vi "Hardware Out - ECS-100X.vi"(11 "RT Data in":T1={"Refs"={"FPGA 1"=refnum, "FPGA 2"=refnum}, "EPT"={"MaxCAD"=0.0, "EPT Sim Enabled"=FALSE, "EPTxData"={"Sync"=FALSE, "CurrentCAD"=0.0, "Speed [RPM]"=0.0, "Config"=FALSE, "Rcvg Primary"=FALSE, "Stall"=FALSE, "Overflow"=FALSE, "Ratio Error"=FALSE, "Pattern Error"=FALSE, "Aux Warning"=FALSE, "Watchdog Error"=FALSE}}, "Raw Inputs"={"NI9752s"=[], "NI9757s"=[], "NI9411s"=[], "NI9220s"=[], "VRHalls"=[]}, "Control Inputs"={"Engine Speed [RPM]"=0.0, "Engine Status"=enum."STALLED", "Load Control \nMode"=enum."High-Idle Governor", "dt(s)"=0.0, "Number of Cylinders"=0, "Engine Displacement [cc]"=0.0, "StoichAFR"=0.0, "Q.LHV Fuel [kJ/kg]"=0.0, "BattV PSU [V]"=0.0, "12V PSU [V]"=0.0, "5V PSU [V]"=0.0, "Pedal Position [%]"=0.0, "Oil Pressure [kPa]"=0.0, "Oil Temp [C]"=0.0, "Oil Level [%]"=0.0, "Engine Coolant Temp (ECT) [C]"=0.0, "Engine Coolant Pressure [kPa]"=0.0, "Rail Pressure [bar]"=0.0, "Fuel Pressure [kPa]"=0.0, "Fuel Temp [C]"=0.0, "Vacuum Pressure [kPa]"=0.0, "Throttle Position [%]"=0.0, "Cam1 Advance [CAD]"=0.0, "Cam2 Advance [CAD]"=0.0, "Cam3 Advance [CAD]"=0.0, "Cam4 Advance [CAD]"=0.0, "CA50 Control Output [CAD]"=[], "CA50 Control Output Valid"=[], "Intake Air Temp (IAT) [C]"=0.0, "Barometric Air Pressure [kPa]"=0.0, "Intake Air Rel. Humidity [%]"=0.0, "Mass Air Flow (MAF) [kg/hr]"=0.0, "Turbo Inlet Air Pressure [kPa]"=0.0, "Turbo Inlet Air Temp [C]"=0.0, "Turbo Outlet Air Pressure [kPa]"=0.0, "Turbo Outlet Air Temp [C]"=0.0, "CAC Outlet Pressure [kPa]"=0.0, "CAC Outlet Temp [C]"=0.0, "Intake Manifold Pressure (MAP) [kPa]"=0.0, "Intake Manifold Temp (MAT) [C]"=0.0, "Exhaust Manifold Pressure [kPa]"=0.0, "Exhaust Manifold Temp [C]"=0.0, "HighP EGR Cooler Outlet Pressure [kPa]"=0.0, "HighP EGR Cooler Outlet Temp [C]"=0.0, "HighP EGR Differential Pressure [kPa]"=0.0, "HighP EGR Valve Position [%]"=0.0, "Turbo Outlet Exhaust Pressure [kPa]"=0.0, "Turbo Outlet Exhaust Temp [C]"=0.0, "VGT Position 1 [%]"=0.0, "VGT Position 2 [%]"=0.0, "Turbo Speed 1 [RPM]"=0.0, "Turbo Speed 2 [RPM]"=0.0, "LowP EGR Differential Pressure [kPa]"=0.0, "LowP EGR Valve Position [%]"=0.0, "UEGO1Lambda"=0.0, "UEGO1_Hot"=FALSE, "UEGO2Lambda"=0.0, "UEGO2_Hot"=FALSE, "Knock Intensity"=[], "Knock"=[]}, "Control Outputs"={"Pedal Desired [%]"=0.0, "MEP Desired [bar]"=0.0, "Fuel Desired [mg/cyc]"=0.0, "Intake MAP Desired [kPa]"=0.0, "Cam1 Advance Setpoint [CAD]"=0.0, "Cam2 Advance Setpoint [CAD]"=0.0, "HighP EGR Position Setpoint [%Open]"=0.0, "LowP EGR Position Setpoint [%Open]"=0.0, "Rail Pressure Setpoint [bar]"=0.0, "Wastegate1 Position Setpoint [%Open]"=0.0, "Wastegate2 Position Setpoint [%Open]"=0.0, "VGT1 Position Setpoint [%Open]"=0.0, "VGT2 Position Setpoint [%Open]"=0.0, "Throttle1 Position Setpoint [%Open]"=0.0, "Throttle2 Position Setpoint [%Open]"=0.0, "TurboBPV Position Setpoint [%Open]"=0.0, "Spark Dwells [msec]"=[], "Spark Timings [DBTDC]"=[], "PFI Quantities [mg/inj]"=[], "PFI Timings [DBTDC]"=[], "DI Quantities [mg/inj]"=[], "DI Timings [DBTDC]"=[]}, "Raw Outputs"={"9751-1"={"DI1"={"Window_Start (DBTDC)"=0.0, "Window_End (DBTDC)"=0.0, "Enable_Inj1"=FALSE, "Duration_Inj1 (msec)"=0.0, "Timing_Inj1 (DBTDC)"=0.0, "Enable_Inj2"=FALSE, "Duration_Inj2 (msec)"=0.0, "Timing_Inj2 (DBTDC)"=0.0, "Enable_Inj3"=FALSE, "Duration_Inj3 (msec)"=0.0, "Timing_Inj3 (DBTDC)"=0.0, "Enable_Inj4"=FALSE, "Duration_Inj4 (msec)"=0.0, "Timing_Inj4 (DBTDC)"=0.0, "Enable_Inj5"=FALSE, "Duration_Inj5 (msec)"=0.0, "Timing_Inj5 (DBTDC)"=0.0}, "DI2"={"Window_Start (DBTDC)"=0.0, "Window_End (DBTDC)"=0.0, "Enable_Inj1"=FALSE, "Duration_Inj1 (msec)"=0.0, "Timing_Inj1 (DBTDC)"=0.0, "Enable_Inj2"=FALSE, "Duration_Inj2 (msec)"=0.0, "Timing_Inj2 (DBTDC)"=0.0, "Enable_Inj3"=FALSE, "Duration_Inj3 (msec)"=0.0, "Timing_Inj3 (DBTDC)"=0.0, "Enable_Inj4"=FALSE, "Duration_Inj4 (msec)"=0.0, "Timing_Inj4 (DBTDC)"=0.0, "Enable_Inj5"=FALSE, "Duration_Inj5 (msec)"=0.0, "Timing_Inj5 (DBTDC)"=0.0}, "DI3"={"Window_Start (DBTDC)"=0.0, "Window_End (DBTDC)"=0.0, "Enable_Inj1"=FALSE, "Duration_Inj1 (msec)"=0.0, "Timing_Inj1 (DBTDC)"=0.0, "Enable_Inj2"=FALSE, "Duration_Inj2 (msec)"=0.0, "Timing_Inj2 (DBTDC)"=0.0, "Enable_Inj3"=FALSE, "Duration_Inj3 (msec)"=0.0, "Timing_Inj3 (DBTDC)"=0.0, "Enable_Inj4"=FALSE, "Duration_Inj4 (msec)"=0.0, "Timing_Inj4 (DBTDC)"=0.0, "Enable_Inj5"=FALSE, "Duration_Inj5 (msec)"=0.0, "Timing_Inj5 (DBTDC)"=0.0}}, "9751-2"={"DI1"={"Window_Start (DBTDC)"=0.0, "Window_End (DBTDC)"=0.0, "Enable_Inj1"=FALSE, "Duration_Inj1 (msec)"=0.0, "Timing_Inj1 (DBTDC)"=0.0, "Enable_Inj2"=FALSE, "Duration_Inj2 (msec)"=0.0, "Timing_Inj2 (DBTDC)"=0.0, "Enable_Inj3"=FALSE, "Duration_Inj3 (msec)"=0.0, "Timing_Inj3 (DBTDC)"=0.0, "Enable_Inj4"=FALSE, "Duration_Inj4 (msec)"=0.0, "Timing_Inj4 (DBTDC)"=0.0, "Enable_Inj5"=FALSE, "Duration_Inj5 (msec)"=0.0, "Timing_Inj5 (DBTDC)"=0.0}, "DI2"={"Window_Start (DBTDC)"=0.0, "Window_End (DBTDC)"=0.0, "Enable_Inj1"=FALSE, "Duration_Inj1 (msec)"=0.0, "Timing_Inj1 (DBTDC)"=0.0, "Enable_Inj2"=FALSE, "Duration_Inj2 (msec)"=0.0, "Timing_Inj2 (DBTDC)"=0.0, "Enable_Inj3"=FALSE, "Duration_Inj3 (msec)"=0.0, "Timing_Inj3 (DBTDC)"=0.0, "Enable_Inj4"=FALSE, "Duration_Inj4 (msec)"=0.0, "Timing_Inj4 (DBTDC)"=0.0, "Enable_Inj5"=FALSE, "Duration_Inj5 (msec)"=0.0, "Timing_Inj5 (DBTDC)"=0.0}, "DI3"={"Window_Start (DBTDC)"=0.0, "Window_End (DBTDC)"=0.0, "Enable_Inj1"=FALSE, "Duration_Inj1 (msec)"=0.0, "Timing_Inj1 (DBTDC)"=0.0, "Enable_Inj2"=FALSE, "Duration_Inj2 (msec)"=0.0, "Timing_Inj2 (DBTDC)"=0.0, "Enable_Inj3"=FALSE, "Duration_Inj3 (msec)"=0.0, "Timing_Inj3 (DBTDC)"=0.0, "Enable_Inj4"=FALSE, "Duration_Inj4 (msec)"=0.0, "Timing_Inj4 (DBTDC)"=0.0, "Enable_Inj5"=FALSE, "Duration_Inj5 (msec)"=0.0, "Timing_Inj5 (DBTDC)"=0.0}}, "9751-3"={"DI1"={"Window_Start (DBTDC)"=0.0, "Window_End (DBTDC)"=0.0, "Enable_Inj1"=FALSE, "Duration_Inj1 (msec)"=0.0, "Timing_Inj1 (DBTDC)"=0.0, "Enable_Inj2"=FALSE, "Duration_Inj2 (msec)"=0.0, "Timing_Inj2 (DBTDC)"=0.0, "Enable_Inj3"=FALSE, "Duration_Inj3 (msec)"=0.0, "Timing_Inj3 (DBTDC)"=0.0, "Enable_Inj4"=FALSE, "Duration_Inj4 (msec)"=0.0, "Timing_Inj4 (DBTDC)"=0.0, "Enable_Inj5"=FALSE, "Duration_Inj5 (msec)"=0.0, "Timing_Inj5 (DBTDC)"=0.0}, "DI2"={"Window_Start (DBTDC)"=0.0, "Window_End (DBTDC)"=0.0, "Enable_Inj1"=FALSE, "Duration_Inj1 (msec)"=0.0, "Timing_Inj1 (DBTDC)"=0.0, "Enable_Inj2"=FALSE, "Duration_Inj2 (msec)"=0.0, "Timing_Inj2 (DBTDC)"=0.0, "Enable_Inj3"=FALSE, "Duration_Inj3 (msec)"=0.0, "Timing_Inj3 (DBTDC)"=0.0, "Enable_Inj4"=FALSE, "Duration_Inj4 (msec)"=0.0, "Timing_Inj4 (DBTDC)"=0.0, "Enable_Inj5"=FALSE, "Duration_Inj5 (msec)"=0.0, "Timing_Inj5 (DBTDC)"=0.0}, "DI3"={"Window_Start (DBTDC)"=0.0, "Window_End (DBTDC)"=0.0, "Enable_Inj1"=FALSE, "Duration_Inj1 (msec)"=0.0, "Timing_Inj1 (DBTDC)"=0.0, "Enable_Inj2"=FALSE, "Duration_Inj2 (msec)"=0.0, "Timing_Inj2 (DBTDC)"=0.0, "Enable_Inj3"=FALSE, "Duration_Inj3 (msec)"=0.0, "Timing_Inj3 (DBTDC)"=0.0, "Enable_Inj4"=FALSE, "Duration_Inj4 (msec)"=0.0, "Timing_Inj4 (DBTDC)"=0.0, "Enable_Inj5"=FALSE, "Duration_Inj5 (msec)"=0.0, "Timing_Inj5 (DBTDC)"=0.0}}, "9751-4"={"DI1"={"Window_Start (DBTDC)"=0.0, "Window_End (DBTDC)"=0.0, "Enable_Inj1"=FALSE, "Duration_Inj1 (msec)"=0.0, "Timing_Inj1 (DBTDC)"=0.0, "Enable_Inj2"=FALSE, "Duration_Inj2 (msec)"=0.0, "Timing_Inj2 (DBTDC)"=0.0, "Enable_Inj3"=FALSE, "Duration_Inj3 (msec)"=0.0, "Timing_Inj3 (DBTDC)"=0.0, "Enable_Inj4"=FALSE, "Duration_Inj4 (msec)"=0.0, "Timing_Inj4 (DBTDC)"=0.0, "Enable_Inj5"=FALSE, "Duration_Inj5 (msec)"=0.0, "Timing_Inj5 (DBTDC)"=0.0}, "DI2"={"Window_Start (DBTDC)"=0.0, "Window_End (DBTDC)"=0.0, "Enable_Inj1"=FALSE, "Duration_Inj1 (msec)"=0.0, "Timing_Inj1 (DBTDC)"=0.0, "Enable_Inj2"=FALSE, "Duration_Inj2 (msec)"=0.0, "Timing_Inj2 (DBTDC)"=0.0, "Enable_Inj3"=FALSE, "Duration_Inj3 (msec)"=0.0, "Timing_Inj3 (DBTDC)"=0.0, "Enable_Inj4"=FALSE, "Duration_Inj4 (msec)"=0.0, "Timing_Inj4 (DBTDC)"=0.0, "Enable_Inj5"=FALSE, "Duration_Inj5 (msec)"=0.0, "Timing_Inj5 (DBTDC)"=0.0}, "DI3"={"Window_Start (DBTDC)"=0.0, "Window_End (DBTDC)"=0.0, "Enable_Inj1"=FALSE, "Duration_Inj1 (msec)"=0.0, "Timing_Inj1 (DBTDC)"=0.0, "Enable_Inj2"=FALSE, "Duration_Inj2 (msec)"=0.0, "Timing_Inj2 (DBTDC)"=0.0, "Enable_Inj3"=FALSE, "Duration_Inj3 (msec)"=0.0, "Timing_Inj3 (DBTDC)"=0.0, "Enable_Inj4"=FALSE, "Duration_Inj4 (msec)"=0.0, "Timing_Inj4 (DBTDC)"=0.0, "Enable_Inj5"=FALSE, "Duration_Inj5 (msec)"=0.0, "Timing_Inj5 (DBTDC)"=0.0}}, "9754-1"={"ESTTL 1"={"Timing (DBTDC)"=0.0, "Dwell (ms)"=0.0}, "ESTTL 2"={"Timing (DBTDC)"=0.0, "Dwell (ms)"=0.0}, "ESTTL 3"={"Timing (DBTDC)"=0.0, "Dwell (ms)"=0.0}, "ESTTL 4"={"Timing (DBTDC)"=0.0, "Dwell (ms)"=0.0}, "ESTTL 5"={"Timing (DBTDC)"=0.0, "Dwell (ms)"=0.0}, "ESTTL 6"={"Timing (DBTDC)"=0.0, "Dwell (ms)"=0.0}, "ESTTL 7"={"Timing (DBTDC)"=0.0, "Dwell (ms)"=0.0}, "ESTTL 8"={"Timing (DBTDC)"=0.0, "Dwell (ms)"=0.0}}, "9754-2"={"ESTTL 1"={"Timing (DBTDC)"=0.0, "Dwell (ms)"=0.0}, "ESTTL 2"={"Timing (DBTDC)"=0.0, "Dwell (ms)"=0.0}, "ESTTL 3"={"Timing (DBTDC)"=0.0, "Dwell (ms)"=0.0}, "ESTTL 4"={"Timing (DBTDC)"=0.0, "Dwell (ms)"=0.0}, "ESTTL 5"={"Timing (DBTDC)"=0.0, "Dwell (ms)"=0.0}, "ESTTL 6"={"Timing (DBTDC)"=0.0, "Dwell (ms)"=0.0}, "ESTTL 7"={"Timing (DBTDC)"=0.0, "Dwell (ms)"=0.0}, "ESTTL 8"={"Timing (DBTDC)"=0.0, "Dwell (ms)"=0.0}}, "9758-1"={"LS 1"={"Enable"=FALSE, "Freq [Hz]"=0.0, "DutyCyc [%]"=0.0}, "LS 2"={"Enable"=FALSE, "Freq [Hz]"=0.0, "DutyCyc [%]"=0.0}, "LS 3"={"Enable"=FALSE, "Freq [Hz]"=0.0, "DutyCyc [%]"=0.0}, "LS 4"={"Enable"=FALSE, "Freq [Hz]"=0.0, "DutyCyc [%]"=0.0}, "PFI 1"={"Position Mode"=FALSE, "Timing (DBTDC)"=0.0, "Pulse Width (ms)"=0.0}, "PFI 2"={"Position Mode"=FALSE, "Timing (DBTDC)"=0.0, "Pulse Width (ms)"=0.0}, "PFI 3"={"Position Mode"=FALSE, "Timing (DBTDC)"=0.0, "Pulse Width (ms)"=0.0}, "PFI 4"={"Position Mode"=FALSE, "Timing (DBTDC)"=0.0, "Pulse Width (ms)"=0.0}}, "9758-2"={"LS 1"={"Enable"=FALSE, "Freq [Hz]"=0.0, "DutyCyc [%]"=0.0}, "LS 2"={"Enable"=FALSE, "Freq [Hz]"=0.0, "DutyCyc [%]"=0.0}, "LS 3"={"Enable"=FALSE, "Freq [Hz]"=0.0, "DutyCyc [%]"=0.0}, "LS 4"={"Enable"=FALSE, "Freq [Hz]"=0.0, "DutyCyc [%]"=0.0}, "PFI 1"={"Position Mode"=FALSE, "Timing (DBTDC)"=0.0, "Pulse Width (ms)"=0.0}, "PFI 2"={"Position Mode"=FALSE, "Timing (DBTDC)"=0.0, "Pulse Width (ms)"=0.0}, "PFI 3"={"Position Mode"=FALSE, "Timing (DBTDC)"=0.0, "Pulse Width (ms)"=0.0}, "PFI 4"={"Position Mode"=FALSE, "Timing (DBTDC)"=0.0, "Pulse Width (ms)"=0.0}}, "9759-1"={"THR1-1 DC [%]"=0.0, "THR1-1 Setpoint [% Open]"=0.0, "THR1-2 DC [%]"=0.0, "THR1-2 Setpoint [% Open]"=0.0}}} {"Control Inputs"."Knock Intensity" format="%.2f"; "Control Inputs"."CA50 Control Output [CAD]" format="%.2f"; "Control Inputs"."Exhaust Manifold Temp [C]" format="%#_6f"; "Control Inputs"."UEGO2Lambda" format="%.2f"; "Control Inputs"."Intake Manifold Temp (MAT) [C]" format="%#_6f"; "Control Inputs"."UEGO1Lambda" format="%.2f"}) -> (3 "RT Data out":T1={"Refs"={"FPGA 1"=refnum, "FPGA 2"=refnum}, "EPT"={"MaxCAD"=0.0, "EPT Sim Enabled"=FALSE, "EPTxData"={"Sync"=FALSE, "CurrentCAD"=0.0, "Speed [RPM]"=0.0, "Config"=FALSE, "Rcvg Primary"=FALSE, "Stall"=FALSE, "Overflow"=FALSE, "Ratio Error"=FALSE, "Pattern Error"=FALSE, "Aux Warning"=FALSE, "Watchdog Error"=FALSE}}, "Raw Inputs"={"NI9752s"=[], "NI9757s"=[], "NI9411s"=[], "NI9220s"=[], "VRHalls"=[]}, "Control Inputs"={"Engine Speed [RPM]"=0.0, "Engine Status"=enum."STALLED", "Load Control \nMode"=enum."High-Idle Governor", "dt(s)"=0.0, "Number of Cylinders"=0, "Engine Displacement [cc]"=0.0, "StoichAFR"=0.0, "Q.LHV Fuel [kJ/kg]"=0.0, "BattV PSU [V]"=0.0, "12V PSU [V]"=0.0, "5V PSU [V]"=0.0, "Pedal Position [%]"=0.0, "Oil Pressure [kPa]"=0.0, "Oil Temp [C]"=0.0, "Oil Level [%]"=0.0, "Engine Coolant Temp (ECT) [C]"=0.0, "Engine Coolant Pressure [kPa]"=0.0, "Rail Pressure [bar]"=0.0, "Fuel Pressure [kPa]"=0.0, "Fuel Temp [C]"=0.0, "Vacuum Pressure [kPa]"=0.0, "Throttle Position [%]"=0.0, "Cam1 Advance [CAD]"=0.0, "Cam2 Advance [CAD]"=0.0, "Cam3 Advance [CAD]"=0.0, "Cam4 Advance [CAD]"=0.0, "CA50 Control Output [CAD]"=[], "CA50 Control Output Valid"=[], "Intake Air Temp (IAT) [C]"=0.0, "Barometric Air Pressure [kPa]"=0.0, "Intake Air Rel. Humidity [%]"=0.0, "Mass Air Flow (MAF) [kg/hr]"=0.0, "Turbo Inlet Air Pressure [kPa]"=0.0, "Turbo Inlet Air Temp [C]"=0.0, "Turbo Outlet Air Pressure [kPa]"=0.0, "Turbo Outlet Air Temp [C]"=0.0, "CAC Outlet Pressure [kPa]"=0.0, "CAC Outlet Temp [C]"=0.0, "Intake Manifold Pressure (MAP) [kPa]"=0.0, "Intake Manifold Temp (MAT) [C]"=0.0, "Exhaust Manifold Pressure [kPa]"=0.0, "Exhaust Manifold Temp [C]"=0.0, "HighP EGR Cooler Outlet Pressure [kPa]"=0.0, "HighP EGR Cooler Outlet Temp [C]"=0.0, "HighP EGR Differential Pressure [kPa]"=0.0, "HighP EGR Valve Position [%]"=0.0, "Turbo Outlet Exhaust Pressure [kPa]"=0.0, "Turbo Outlet Exhaust Temp [C]"=0.0, "VGT Position 1 [%]"=0.0, "VGT Position 2 [%]"=0.0, "Turbo Speed 1 [RPM]"=0.0, "Turbo Speed 2 [RPM]"=0.0, "LowP EGR Differential Pressure [kPa]"=0.0, "LowP EGR Valve Position [%]"=0.0, "UEGO1Lambda"=0.0, "UEGO1_Hot"=FALSE, "UEGO2Lambda"=0.0, "UEGO2_Hot"=FALSE, "Knock Intensity"=[], "Knock"=[]}, "Control Outputs"={"Pedal Desired [%]"=0.0, "MEP Desired [bar]"=0.0, "Fuel Desired [mg/cyc]"=0.0, "Intake MAP Desired [kPa]"=0.0, "Cam1 Advance Setpoint [CAD]"=0.0, "Cam2 Advance Setpoint [CAD]"=0.0, "HighP EGR Position Setpoint [%Open]"=0.0, "LowP EGR Position Setpoint [%Open]"=0.0, "Rail Pressure Setpoint [bar]"=0.0, "Wastegate1 Position Setpoint [%Open]"=0.0, "Wastegate2 Position Setpoint [%Open]"=0.0, "VGT1 Position Setpoint [%Open]"=0.0, "VGT2 Position Setpoint [%Open]"=0.0, "Throttle1 Position Setpoint [%Open]"=0.0, "Throttle2 Position Setpoint [%Open]"=0.0, "TurboBPV Position Setpoint [%Open]"=0.0, "Spark Dwells [msec]"=[], "Spark Timings [DBTDC]"=[], "PFI Quantities [mg/inj]"=[], "PFI Timings [DBTDC]"=[], "DI Quantities [mg/inj]"=[], "DI Timings [DBTDC]"=[]}, "Raw Outputs"={"9751-1"={"DI1"={"Window_Start (DBTDC)"=0.0, "Window_End (DBTDC)"=0.0, "Enable_Inj1"=FALSE, "Duration_Inj1 (msec)"=0.0, "Timing_Inj1 (DBTDC)"=0.0, "Enable_Inj2"=FALSE, "Duration_Inj2 (msec)"=0.0, "Timing_Inj2 (DBTDC)"=0.0, "Enable_Inj3"=FALSE, "Duration_Inj3 (msec)"=0.0, "Timing_Inj3 (DBTDC)"=0.0, "Enable_Inj4"=FALSE, "Duration_Inj4 (msec)"=0.0, "Timing_Inj4 (DBTDC)"=0.0, "Enable_Inj5"=FALSE, "Duration_Inj5 (msec)"=0.0, "Timing_Inj5 (DBTDC)"=0.0}, "DI2"={"Window_Start (DBTDC)"=0.0, "Window_End (DBTDC)"=0.0, "Enable_Inj1"=FALSE, "Duration_Inj1 (msec)"=0.0, "Timing_Inj1 (DBTDC)"=0.0, "Enable_Inj2"=FALSE, "Duration_Inj2 (msec)"=0.0, "Timing_Inj2 (DBTDC)"=0.0, "Enable_Inj3"=FALSE, "Duration_Inj3 (msec)"=0.0, "Timing_Inj3 (DBTDC)"=0.0, "Enable_Inj4"=FALSE, "Duration_Inj4 (msec)"=0.0, "Timing_Inj4 (DBTDC)"=0.0, "Enable_Inj5"=FALSE, "Duration_Inj5 (msec)"=0.0, "Timing_Inj5 (DBTDC)"=0.0}, "DI3"={"Window_Start (DBTDC)"=0.0, "Window_End (DBTDC)"=0.0, "Enable_Inj1"=FALSE, "Duration_Inj1 (msec)"=0.0, "Timing_Inj1 (DBTDC)"=0.0, "Enable_Inj2"=FALSE, "Duration_Inj2 (msec)"=0.0, "Timing_Inj2 (DBTDC)"=0.0, "Enable_Inj3"=FALSE, "Duration_Inj3 (msec)"=0.0, "Timing_Inj3 (DBTDC)"=0.0, "Enable_Inj4"=FALSE, "Duration_Inj4 (msec)"=0.0, "Timing_Inj4 (DBTDC)"=0.0, "Enable_Inj5"=FALSE, "Duration_Inj5 (msec)"=0.0, "Timing_Inj5 (DBTDC)"=0.0}}, "9751-2"={"DI1"={"Window_Start (DBTDC)"=0.0, "Window_End (DBTDC)"=0.0, "Enable_Inj1"=FALSE, "Duration_Inj1 (msec)"=0.0, "Timing_Inj1 (DBTDC)"=0.0, "Enable_Inj2"=FALSE, "Duration_Inj2 (msec)"=0.0, "Timing_Inj2 (DBTDC)"=0.0, "Enable_Inj3"=FALSE, "Duration_Inj3 (msec)"=0.0, "Timing_Inj3 (DBTDC)"=0.0, "Enable_Inj4"=FALSE, "Duration_Inj4 (msec)"=0.0, "Timing_Inj4 (DBTDC)"=0.0, "Enable_Inj5"=FALSE, "Duration_Inj5 (msec)"=0.0, "Timing_Inj5 (DBTDC)"=0.0}, "DI2"={"Window_Start (DBTDC)"=0.0, "Window_End (DBTDC)"=0.0, "Enable_Inj1"=FALSE, "Duration_Inj1 (msec)"=0.0, "Timing_Inj1 (DBTDC)"=0.0, "Enable_Inj2"=FALSE, "Duration_Inj2 (msec)"=0.0, "Timing_Inj2 (DBTDC)"=0.0, "Enable_Inj3"=FALSE, "Duration_Inj3 (msec)"=0.0, "Timing_Inj3 (DBTDC)"=0.0, "Enable_Inj4"=FALSE, "Duration_Inj4 (msec)"=0.0, "Timing_Inj4 (DBTDC)"=0.0, "Enable_Inj5"=FALSE, "Duration_Inj5 (msec)"=0.0, "Timing_Inj5 (DBTDC)"=0.0}, "DI3"={"Window_Start (DBTDC)"=0.0, "Window_End (DBTDC)"=0.0, "Enable_Inj1"=FALSE, "Duration_Inj1 (msec)"=0.0, "Timing_Inj1 (DBTDC)"=0.0, "Enable_Inj2"=FALSE, "Duration_Inj2 (msec)"=0.0, "Timing_Inj2 (DBTDC)"=0.0, "Enable_Inj3"=FALSE, "Duration_Inj3 (msec)"=0.0, "Timing_Inj3 (DBTDC)"=0.0, "Enable_Inj4"=FALSE, "Duration_Inj4 (msec)"=0.0, "Timing_Inj4 (DBTDC)"=0.0, "Enable_Inj5"=FALSE, "Duration_Inj5 (msec)"=0.0, "Timing_Inj5 (DBTDC)"=0.0}}, "9751-3"={"DI1"={"Window_Start (DBTDC)"=0.0, "Window_End (DBTDC)"=0.0, "Enable_Inj1"=FALSE, "Duration_Inj1 (msec)"=0.0, "Timing_Inj1 (DBTDC)"=0.0, "Enable_Inj2"=FALSE, "Duration_Inj2 (msec)"=0.0, "Timing_Inj2 (DBTDC)"=0.0, "Enable_Inj3"=FALSE, "Duration_Inj3 (msec)"=0.0, "Timing_Inj3 (DBTDC)"=0.0, "Enable_Inj4"=FALSE, "Duration_Inj4 (msec)"=0.0, "Timing_Inj4 (DBTDC)"=0.0, "Enable_Inj5"=FALSE, "Duration_Inj5 (msec)"=0.0, "Timing_Inj5 (DBTDC)"=0.0}, "DI2"={"Window_Start (DBTDC)"=0.0, "Window_End (DBTDC)"=0.0, "Enable_Inj1"=FALSE, "Duration_Inj1 (msec)"=0.0, "Timing_Inj1 (DBTDC)"=0.0, "Enable_Inj2"=FALSE, "Duration_Inj2 (msec)"=0.0, "Timing_Inj2 (DBTDC)"=0.0, "Enable_Inj3"=FALSE, "Duration_Inj3 (msec)"=0.0, "Timing_Inj3 (DBTDC)"=0.0, "Enable_Inj4"=FALSE, "Duration_Inj4 (msec)"=0.0, "Timing_Inj4 (DBTDC)"=0.0, "Enable_Inj5"=FALSE, "Duration_Inj5 (msec)"=0.0, "Timing_Inj5 (DBTDC)"=0.0}, "DI3"={"Window_Start (DBTDC)"=0.0, "Window_End (DBTDC)"=0.0, "Enable_Inj1"=FALSE, "Duration_Inj1 (msec)"=0.0, "Timing_Inj1 (DBTDC)"=0.0, "Enable_Inj2"=FALSE, "Duration_Inj2 (msec)"=0.0, "Timing_Inj2 (DBTDC)"=0.0, "Enable_Inj3"=FALSE, "Duration_Inj3 (msec)"=0.0, "Timing_Inj3 (DBTDC)"=0.0, "Enable_Inj4"=FALSE, "Duration_Inj4 (msec)"=0.0, "Timing_Inj4 (DBTDC)"=0.0, "Enable_Inj5"=FALSE, "Duration_Inj5 (msec)"=0.0, "Timing_Inj5 (DBTDC)"=0.0}}, "9751-4"={"DI1"={"Window_Start (DBTDC)"=0.0, "Window_End (DBTDC)"=0.0, "Enable_Inj1"=FALSE, "Duration_Inj1 (msec)"=0.0, "Timing_Inj1 (DBTDC)"=0.0, "Enable_Inj2"=FALSE, "Duration_Inj2 (msec)"=0.0, "Timing_Inj2 (DBTDC)"=0.0, "Enable_Inj3"=FALSE, "Duration_Inj3 (msec)"=0.0, "Timing_Inj3 (DBTDC)"=0.0, "Enable_Inj4"=FALSE, "Duration_Inj4 (msec)"=0.0, "Timing_Inj4 (DBTDC)"=0.0, "Enable_Inj5"=FALSE, "Duration_Inj5 (msec)"=0.0, "Timing_Inj5 (DBTDC)"=0.0}, "DI2"={"Window_Start (DBTDC)"=0.0, "Window_End (DBTDC)"=0.0, "Enable_Inj1"=FALSE, "Duration_Inj1 (msec)"=0.0, "Timing_Inj1 (DBTDC)"=0.0, "Enable_Inj2"=FALSE, "Duration_Inj2 (msec)"=0.0, "Timing_Inj2 (DBTDC)"=0.0, "Enable_Inj3"=FALSE, "Duration_Inj3 (msec)"=0.0, "Timing_Inj3 (DBTDC)"=0.0, "Enable_Inj4"=FALSE, "Duration_Inj4 (msec)"=0.0, "Timing_Inj4 (DBTDC)"=0.0, "Enable_Inj5"=FALSE, "Duration_Inj5 (msec)"=0.0, "Timing_Inj5 (DBTDC)"=0.0}, "DI3"={"Window_Start (DBTDC)"=0.0, "Window_End (DBTDC)"=0.0, "Enable_Inj1"=FALSE, "Duration_Inj1 (msec)"=0.0, "Timing_Inj1 (DBTDC)"=0.0, "Enable_Inj2"=FALSE, "Duration_Inj2 (msec)"=0.0, "Timing_Inj2 (DBTDC)"=0.0, "Enable_Inj3"=FALSE, "Duration_Inj3 (msec)"=0.0, "Timing_Inj3 (DBTDC)"=0.0, "Enable_Inj4"=FALSE, "Duration_Inj4 (msec)"=0.0, "Timing_Inj4 (DBTDC)"=0.0, "Enable_Inj5"=FALSE, "Duration_Inj5 (msec)"=0.0, "Timing_Inj5 (DBTDC)"=0.0}}, "9754-1"={"ESTTL 1"={"Timing (DBTDC)"=0.0, "Dwell (ms)"=0.0}, "ESTTL 2"={"Timing (DBTDC)"=0.0, "Dwell (ms)"=0.0}, "ESTTL 3"={"Timing (DBTDC)"=0.0, "Dwell (ms)"=0.0}, "ESTTL 4"={"Timing (DBTDC)"=0.0, "Dwell (ms)"=0.0}, "ESTTL 5"={"Timing (DBTDC)"=0.0, "Dwell (ms)"=0.0}, "ESTTL 6"={"Timing (DBTDC)"=0.0, "Dwell (ms)"=0.0}, "ESTTL 7"={"Timing (DBTDC)"=0.0, "Dwell (ms)"=0.0}, "ESTTL 8"={"Timing (DBTDC)"=0.0, "Dwell (ms)"=0.0}}, "9754-2"={"ESTTL 1"={"Timing (DBTDC)"=0.0, "Dwell (ms)"=0.0}, "ESTTL 2"={"Timing (DBTDC)"=0.0, "Dwell (ms)"=0.0}, "ESTTL 3"={"Timing (DBTDC)"=0.0, "Dwell (ms)"=0.0}, "ESTTL 4"={"Timing (DBTDC)"=0.0, "Dwell (ms)"=0.0}, "ESTTL 5"={"Timing (DBTDC)"=0.0, "Dwell (ms)"=0.0}, "ESTTL 6"={"Timing (DBTDC)"=0.0, "Dwell (ms)"=0.0}, "ESTTL 7"={"Timing (DBTDC)"=0.0, "Dwell (ms)"=0.0}, "ESTTL 8"={"Timing (DBTDC)"=0.0, "Dwell (ms)"=0.0}}, "9758-1"={"LS 1"={"Enable"=FALSE, "Freq [Hz]"=0.0, "DutyCyc [%]"=0.0}, "LS 2"={"Enable"=FALSE, "Freq [Hz]"=0.0, "DutyCyc [%]"=0.0}, "LS 3"={"Enable"=FALSE, "Freq [Hz]"=0.0, "DutyCyc [%]"=0.0}, "LS 4"={"Enable"=FALSE, "Freq [Hz]"=0.0, "DutyCyc [%]"=0.0}, "PFI 1"={"Position Mode"=FALSE, "Timing (DBTDC)"=0.0, "Pulse Width (ms)"=0.0}, "PFI 2"={"Position Mode"=FALSE, "Timing (DBTDC)"=0.0, "Pulse Width (ms)"=0.0}, "PFI 3"={"Position Mode"=FALSE, "Timing (DBTDC)"=0.0, "Pulse Width (ms)"=0.0}, "PFI 4"={"Position Mode"=FALSE, "Timing (DBTDC)"=0.0, "Pulse Width (ms)"=0.0}}, "9758-2"={"LS 1"={"Enable"=FALSE, "Freq [Hz]"=0.0, "DutyCyc [%]"=0.0}, "LS 2"={"Enable"=FALSE, "Freq [Hz]"=0.0, "DutyCyc [%]"=0.0}, "LS 3"={"Enable"=FALSE, "Freq [Hz]"=0.0, "DutyCyc [%]"=0.0}, "LS 4"={"Enable"=FALSE, "Freq [Hz]"=0.0, "DutyCyc [%]"=0.0}, "PFI 1"={"Position Mode"=FALSE, "Timing (DBTDC)"=0.0, "Pulse Width (ms)"=0.0}, "PFI 2"={"Position Mode"=FALSE, "Timing (DBTDC)"=0.0, "Pulse Width (ms)"=0.0}, "PFI 3"={"Position Mode"=FALSE, "Timing (DBTDC)"=0.0, "Pulse Width (ms)"=0.0}, "PFI 4"={"Position Mode"=FALSE, "Timing (DBTDC)"=0.0, "Pulse Width (ms)"=0.0}}, "9759-1"={"THR1-1 DC [%]"=0.0, "THR1-1 Setpoint [% Open]"=0.0, "THR1-2 DC [%]"=0.0, "THR1-2 Setpoint [% Open]"=0.0}}} {"Control Inputs"."Knock Intensity" format="%.2f"; "Control Inputs"."CA50 Control Output [CAD]" format="%.2f"; "Control Inputs"."Exhaust Manifold Temp [C]" format="%#_6f"; "Control Inputs"."UEGO2Lambda" format="%.2f"; "Control Inputs"."Intake Manifold Temp (MAT) [C]" format="%#_6f"; "Control Inputs"."UEGO1Lambda" format="%.2f"})   [LabVIEW 2015, in "ECS-RT.lvlib"]
uses:
  ECS-RT.lvlib
  Typedefs/RT Data.ctl
  Typedefs/FPGA Refs/FPGA Refs.ctl
  Typedefs/FPGA Refs/Generic FPGA Ref.ctl
  Typedefs/EPT/EPT Cluster.ctl
  <vilib>/Powertrain Controls/Device Drivers/Engine Position Tracking/EPTx/RevA/RT/Controls/EPTxData.ctl
  Typedefs/Raw Inputs/Raw Inputs.ctl
  Typedefs/Raw Inputs/NI9752.ctl
  Typedefs/Raw Inputs/PPWData.ctl
  Typedefs/Raw Inputs/NI9757.ctl
  Typedefs/Raw Inputs/NI9411.ctl
  Typedefs/Raw Inputs/NI9220.ctl
  Typedefs/Raw Inputs/VRHall.ctl
  Typedefs/Control Inputs/Control Inputs.ctl
  Typedefs/EPT/Engine Status.ctl
  Typedefs/MISC/Load Control Mode.ctl
  Typedefs/Control Outputs/Control Outputs.ctl
  Typedefs/Control Outputs/Injection Quantity.ctl
  Typedefs/Control Outputs/Injection Timing.ctl
  Typedefs/Raw Outputs/Raw Outputs.ctl
  Typedefs/Raw Outputs/NI9751.ctl
  Typedefs/Raw Outputs/DI.ctl
  Typedefs/Raw Outputs/NI9754.ctl
  Typedefs/Raw Outputs/ESTTL.ctl
  Typedefs/Raw Outputs/NI9758.ctl
  Typedefs/Raw Outputs/LS.ctl
  Typedefs/Raw Outputs/PFI.ctl
  Typedefs/Raw Outputs/NI9759.ctl
  ECS-Shared.lvlib
  <vilib>/Powertrain Controls/Device Drivers/Engine Position Tracking/EPTx/RevA/RT/EPTx - RevA - RT.lvlib
types:
  T1 = typedef "ECS-Shared.lvlib/RT Data.ctl" = cluster{"Refs":T2, "EPT":T4, "Raw Inputs":T6, "Control Inputs":T13, "Control Outputs":T16, "Raw Outputs":T19}
  T2 = typedef "ECS-Shared.lvlib/FPGA Refs.ctl" = cluster{"FPGA 1":T3, "FPGA 2":T3}
  T3 = typedef "ECS-Shared.lvlib/Generic FPGA Ref.ctl" = refnum<k20>
  T4 = typedef "ECS-Shared.lvlib/EPT Cluster.ctl" = cluster{"MaxCAD":sgl, "EPT Sim Enabled":bool, "EPTxData":T5}
  T5 = typedef "EPTx - RevA - RT.lvlib/EPTxData.ctl" = cluster{"Sync":bool, "CurrentCAD":sgl, "Speed [RPM]":sgl, "Config":bool, "Rcvg Primary":bool, "Stall":bool, "Overflow":bool, "Ratio Error":bool, "Pattern Error":bool, "Aux Warning":bool, "Watchdog Error":bool}
  T6 = typedef "ECS-Shared.lvlib/Raw Inputs.ctl" = cluster{"NI9752s":T7[], "NI9757s":T9[], "NI9411s":T10[], "NI9220s":T11[], "VRHalls":T12[]}
  T7 = typedef "ECS-Shared.lvlib/NI9752.ctl" = cluster{"Voltage [V]":sgl[], "Resistance [Ohm]":sgl[], "PPWData VR1":T8, "PPWData VR2":T8, "PPWData Hall1":T8, "PPWData Hall2":T8}
  T8 = typedef "ECS-Shared.lvlib/PPWData.ctl" = cluster{"Period":u32, "PulseWidth":u32, "Stopped":bool}
  T9 = typedef "ECS-Shared.lvlib/NI9757.ctl" = cluster{"UEGO1":cluster{"Lambda":sgl, "Phi":sgl, "AF_Ratio":sgl, "Ip":sgl, "Temp":sgl, "Hot":bool}, "UEGO2":cluster{"Lambda":sgl, "Phi":sgl, "AF_Ratio":sgl, "Ip":sgl, "Temp":sgl, "Hot":bool}, "EGO1":cluster{"Status":enum16{"COLD SENSOR", "FOULED SENSOR", "RICH", "LEAN"}, "SensorV":sgl}, "EGO2":cluster{"Status":enum16{"COLD SENSOR", "FOULED SENSOR", "RICH", "LEAN"}, "SensorV":sgl}, "EGO3":cluster{"Status":enum16{"COLD SENSOR", "FOULED SENSOR", "RICH", "LEAN"}, "SensorV":sgl}, "EGO4":cluster{"Status":enum16{"COLD SENSOR", "FOULED SENSOR", "RICH", "LEAN"}, "SensorV":sgl}}
  T10 = typedef "ECS-Shared.lvlib/NI9411.ctl" = cluster{"PPWData 0":T8, "PPWData 1":T8, "PPWData 2":T8, "PPWData 3":T8, "PPWData 4":T8, "PPWData 5":T8}
  T11 = typedef "ECS-Shared.lvlib/NI9220.ctl" = cluster{"AI 0":sgl, "AI 1":sgl, "AI 2":sgl, "AI 3":sgl, "AI 4":sgl, "AI 5":sgl, "AI 6":sgl, "AI 7":sgl, "AI 8":sgl, "AI 9":sgl, "AI 10":sgl, "AI 11":sgl, "AI 12":sgl, "AI 13":sgl, "AI 14":sgl, "AI 15":sgl}
  T12 = typedef "ECS-Shared.lvlib/VRHall.ctl" = cluster{"PPWData 0":T8, "PPWData 1":T8, "PPWData 2":T8, "PPWData 3":T8, "PPWData 4":T8, "PPWData 5":T8}
  T13 = typedef "ECS-Shared.lvlib/Control Inputs.ctl" = cluster{"Engine Speed [RPM]":sgl, "Engine Status":T14, "Load Control \nMode":T15, "dt(s)":sgl, "Number of Cylinders":u8, "Engine Displacement [cc]":sgl, "StoichAFR":sgl, "Q.LHV Fuel [kJ/kg]":sgl, "BattV PSU [V]":sgl, "12V PSU [V]":sgl, "5V PSU [V]":sgl, "Pedal Position [%]":sgl, "Oil Pressure [kPa]":sgl, "Oil Temp [C]":sgl, "Oil Level [%]":sgl, "Engine Coolant Temp (ECT) [C]":sgl, "Engine Coolant Pressure [kPa]":sgl, "Rail Pressure [bar]":sgl, "Fuel Pressure [kPa]":sgl, "Fuel Temp [C]":sgl, "Vacuum Pressure [kPa]":sgl, "Throttle Position [%]":sgl, "Cam1 Advance [CAD]":sgl, "Cam2 Advance [CAD]":sgl, "Cam3 Advance [CAD]":sgl, "Cam4 Advance [CAD]":sgl, "CA50 Control Output [CAD]":sgl[], "CA50 Control Output Valid":bool[], "Intake Air Temp (IAT) [C]":sgl, "Barometric Air Pressure [kPa]":sgl, "Intake Air Rel. Humidity [%]":sgl, "Mass Air Flow (MAF) [kg/hr]":sgl, "Turbo Inlet Air Pressure [kPa]":sgl, "Turbo Inlet Air Temp [C]":sgl, "Turbo Outlet Air Pressure [kPa]":sgl, "Turbo Outlet Air Temp [C]":sgl, "CAC Outlet Pressure [kPa]":sgl, "CAC Outlet Temp [C]":sgl, "Intake Manifold Pressure (MAP) [kPa]":sgl, "Intake Manifold Temp (MAT) [C]":sgl, "Exhaust Manifold Pressure [kPa]":sgl, "Exhaust Manifold Temp [C]":sgl, "HighP EGR Cooler Outlet Pressure [kPa]":sgl, "HighP EGR Cooler Outlet Temp [C]":sgl, "HighP EGR Differential Pressure [kPa]":sgl, "HighP EGR Valve Position [%]":sgl, "Turbo Outlet Exhaust Pressure [kPa]":sgl, "Turbo Outlet Exhaust Temp [C]":sgl, "VGT Position 1 [%]":sgl, "VGT Position 2 [%]":sgl, "Turbo Speed 1 [RPM]":sgl, "Turbo Speed 2 [RPM]":sgl, "LowP EGR Differential Pressure [kPa]":sgl, "LowP EGR Valve Position [%]":sgl, "UEGO1Lambda":sgl, "UEGO1_Hot":bool, "UEGO2Lambda":sgl, "UEGO2_Hot":bool, "Knock Intensity":sgl[], "Knock":bool[]}
  T14 = typedef "ECS-Shared.lvlib/Engine Status.ctl" = enum16{"OFF", "STALLED", "CRANKING", "RUNNING", "ACCEL", "DECEL", "SAFE"}
  T15 = typedef "ECS-Shared.lvlib/Load Control Mode.ctl" = enum16{"No Governor", "Low-Idle Governor", "High-Idle Governor"}
  T16 = typedef "ECS-Shared.lvlib/Control Outputs.ctl" = cluster{"Pedal Desired [%]":sgl, "MEP Desired [bar]":sgl, "Fuel Desired [mg/cyc]":sgl, "Intake MAP Desired [kPa]":sgl, "Cam1 Advance Setpoint [CAD]":sgl, "Cam2 Advance Setpoint [CAD]":sgl, "HighP EGR Position Setpoint [%Open]":sgl, "LowP EGR Position Setpoint [%Open]":sgl, "Rail Pressure Setpoint [bar]":sgl, "Wastegate1 Position Setpoint [%Open]":sgl, "Wastegate2 Position Setpoint [%Open]":sgl, "VGT1 Position Setpoint [%Open]":sgl, "VGT2 Position Setpoint [%Open]":sgl, "Throttle1 Position Setpoint [%Open]":sgl, "Throttle2 Position Setpoint [%Open]":sgl, "TurboBPV Position Setpoint [%Open]":sgl, "Spark Dwells [msec]":sgl[], "Spark Timings [DBTDC]":sgl[], "PFI Quantities [mg/inj]":sgl[], "PFI Timings [DBTDC]":sgl[], "DI Quantities [mg/inj]":T17[], "DI Timings [DBTDC]":T18[]}
  T17 = typedef "ECS-Shared.lvlib/Injection Quantity.ctl" = cluster{"Pilot1Quantity [mg/inj]":sgl, "Pilot2Quantity [mg/inj]":sgl, "MainQuantity [mg/inj]":sgl, "Post1Quantity [mg/inj]":sgl, "Post2Quantity [mg/inj]":sgl}
  T18 = typedef "ECS-Shared.lvlib/Injection Timing.ctl" = cluster{"Pilot1SOI [DBTDC]":sgl, "Pilot2SOI [DBTDC]":sgl, "MainSOI [DBTDC]":sgl, "Post1SOI [DBTDC]":sgl, "Post2SOI [DBTDC]":sgl}
  T19 = typedef "ECS-Shared.lvlib/Raw Outputs.ctl" = cluster{"9751-1":T20, "9751-2":T20, "9751-3":T20, "9751-4":T20, "9754-1":T22, "9754-2":T22, "9758-1":T24, "9758-2":T24, "9759-1":T27}
  T20 = typedef "ECS-Shared.lvlib/NI9751.ctl" = cluster{"DI1":T21, "DI2":T21, "DI3":T21}
  T21 = typedef "ECS-Shared.lvlib/DI.ctl" = cluster{"Window_Start (DBTDC)":sgl, "Window_End (DBTDC)":sgl, "Enable_Inj1":bool, "Duration_Inj1 (msec)":sgl, "Timing_Inj1 (DBTDC)":sgl, "Enable_Inj2":bool, "Duration_Inj2 (msec)":sgl, "Timing_Inj2 (DBTDC)":sgl, "Enable_Inj3":bool, "Duration_Inj3 (msec)":sgl, "Timing_Inj3 (DBTDC)":sgl, "Enable_Inj4":bool, "Duration_Inj4 (msec)":sgl, "Timing_Inj4 (DBTDC)":sgl, "Enable_Inj5":bool, "Duration_Inj5 (msec)":sgl, "Timing_Inj5 (DBTDC)":sgl}
  T22 = typedef "ECS-Shared.lvlib/NI9754.ctl" = cluster{"ESTTL 1":T23, "ESTTL 2":T23, "ESTTL 3":T23, "ESTTL 4":T23, "ESTTL 5":T23, "ESTTL 6":T23, "ESTTL 7":T23, "ESTTL 8":T23}
  T23 = typedef "ECS-Shared.lvlib/ESTTL.ctl" = cluster{"Timing (DBTDC)":sgl, "Dwell (ms)":sgl}
  T24 = typedef "ECS-Shared.lvlib/NI9758.ctl" = cluster{"LS 1":T25, "LS 2":T25, "LS 3":T25, "LS 4":T25, "PFI 1":T26, "PFI 2":T26, "PFI 3":T26, "PFI 4":T26}
  T25 = typedef "ECS-Shared.lvlib/LS.ctl" = cluster{"Enable":bool, "Freq [Hz]":sgl, "DutyCyc [%]":sgl}
  T26 = typedef "ECS-Shared.lvlib/PFI.ctl" = cluster{"Position Mode":bool, "Timing (DBTDC)":sgl, "Pulse Width (ms)":sgl}
  T27 = typedef "ECS-Shared.lvlib/NI9759.ctl" = cluster{"THR1-1 DC [%]":sgl, "THR1-1 Setpoint [% Open]":sgl, "THR1-2 DC [%]":sgl, "THR1-2 Setpoint [% Open]":sgl}
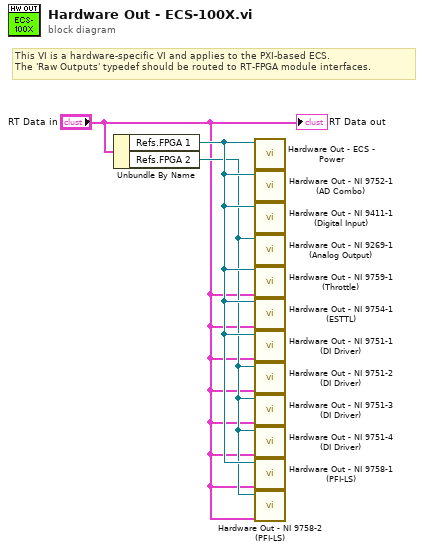
[diagram p0: block diagram]
diagram:
  # "This VI is a hardware-specific VI and applies to the PXI-based ECS.  \nThe 'Raw Outputs' typedef should be routed to RT-FPGA module interfaces."
  n1 = Unbundle By Name("RT Data in") -> ("Refs.FPGA 1"=w3:T3, "Refs.FPGA 2"=w2:T3)
  n2 = call "Hardware Out - ECS - Power.vi"("FPGA Ref"=w3) -> ()  [unwired: 11 in]
  n3 = call "Hardware Out - NI 9752-1 (AD Combo).vi"("FPGA Ref"=w3) -> ()  [unwired: 11 in]
  n4 = call "Hardware Out - NI 9411-1 (Digital Input).vi"("FPGA Ref"=w3) -> ()  [unwired: 11 in]
  n5 = call "Hardware Out - NI 9269-1 (Analog Output).vi"("FPGA Ref"=w2) -> ()  [unwired: 11 in]
  n6 = call "Hardware Out - NI 9759-1 (Throttle).vi"("FPGA Ref"=w3, "RT Data in"="RT Data in") -> ()  [unwired: 14 in]
  n7 = call "Hardware Out - NI 9754-1 (ESTTL).vi"("FPGA Ref"=w3, "RT Data in"="RT Data in") -> ()  [unwired: 14 in]
  n8 = call "Hardware Out - NI 9751-1 (DI Driver).vi"("RT Data in"="RT Data in", "FPGA Ref"=w3) -> ()  [unwired: 10 in]
  n9 = call "Hardware Out - NI 9751-2 (DI Driver).vi"("RT Data in"="RT Data in", "FPGA Ref"=w2) -> ()  [unwired: 10 in]
  n10 = call "Hardware Out - NI 9751-3 (DI Driver).vi"("RT Data in"="RT Data in", "FPGA Ref"=w2) -> ()  [unwired: 10 in]
  n11 = call "Hardware Out - NI 9751-4 (DI Driver).vi"("RT Data in"="RT Data in", "FPGA Ref"=w2) -> ()  [unwired: 10 in]
  n12 = call "Hardware Out - NI 9758-1 (PFI-LS).vi"("RT Data in"="RT Data in", "FPGA Ref"=w3) -> ()  [unwired: 10 in]
  n13 = call "Hardware Out - NI 9758-2 (PFI-LS).vi"("RT Data in"="RT Data in", "FPGA Ref"=w2) -> ()  [unwired: 10 in]
  "RT Data out" <- "RT Data in"
